vi "Get Description.vi"(11 "Mocha in":refnum<class "Milk.lvclass">) -> (2 "Description":string, 3 "Mocha out":refnum<class "Milk.lvclass">)   [LabVIEW 2011, in "Milk.lvclass"]
uses:
  Milk.lvclass
  Milk.lvclass/Milk.ctl
  Beverage/Beverage.lvclass
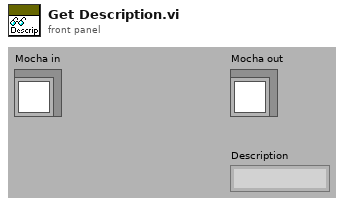
[diagram p1: front panel]
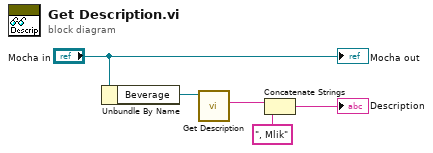
[diagram p0: block diagram]
diagram:
  n1 = Unbundle By Name("Mocha in") -> ("Beverage"=w4:refnum<class "Beverage.lvclass">)
  n2 = call-dynamic "Get Description.vi"("Beverage in"=w4) -> ("Description"=w3:string)  [unwired: 9 in, 1 out]
  n3 = Concatenate Strings(w3, ", Mlik" ("string")) -> (→"Description":string)
  "Mocha out" <- "Mocha in"
